vi "INI Input Clusters.vi"() -> (0 "File output directories":T2={"Archive Location"=path "", "Archive Location 2"=path "<Not A Path>", "OutPut Path"=path "", "Directory(s) To Scan Files"=[]}, 1 "FTP CRED Cluster":T4={"Host"="", "UserName"="", "PassWord"="", "FTP File Path"="", "FTP Timeout (S)"=60, "Active or Passive"=FALSE, "ASCII or Binary"=FALSE} {"FTP Timeout (S)" min=0 max=300 step=1}, 2 "Email Notification Cluster":T3={"Mail Server"="", "Return Address"="", "Email User Name"="", "Password"="", "Ping Address 1"="10.0.0.40", "Ping Address 2"="google.com", "Ping Address FTP Host"="web1026.ixwebhosting.com", "Ping address 1"=FALSE, "Ping address 2"=FALSE, "Ping FTP Host"=FALSE}, 3 "Email Recipiant List":string[](array[string]), 4 "error out":errorcluster, 5 "time stamp":timestamp, 6 "Site ID":string, 7 "File Management cluster":T1, 8 "Auto FTP":bool, 9 "Auto Archive":bool, 11 "hours old date mod(hours)":u8=2)   [LabVIEW 2011]
uses:
  Controls/FTP Credintials.ctl
  Controls/Ping address and email notify.ctl
  Controls/File Path directories.ctl
  Controls/File Management.ctl
  <vilib>/Utility/sysdir.llb/System Directory Type.ctl
  <vilib>/Utility/config.llb/Read Key (String).vi
  <vilib>/Utility/config.llb/Read Key (Boolean).vi
  <vilib>/Utility/config.llb/Read Key (Path).vi
  <vilib>/Utility/config.llb/Read Key (I32).vi
  <vilib>/Utility/config.llb/Read Key (U32).vi
  <vilib>/Utility/config.llb/NI_LVConfig.lvlib
panel:
  # "File Handling Method"
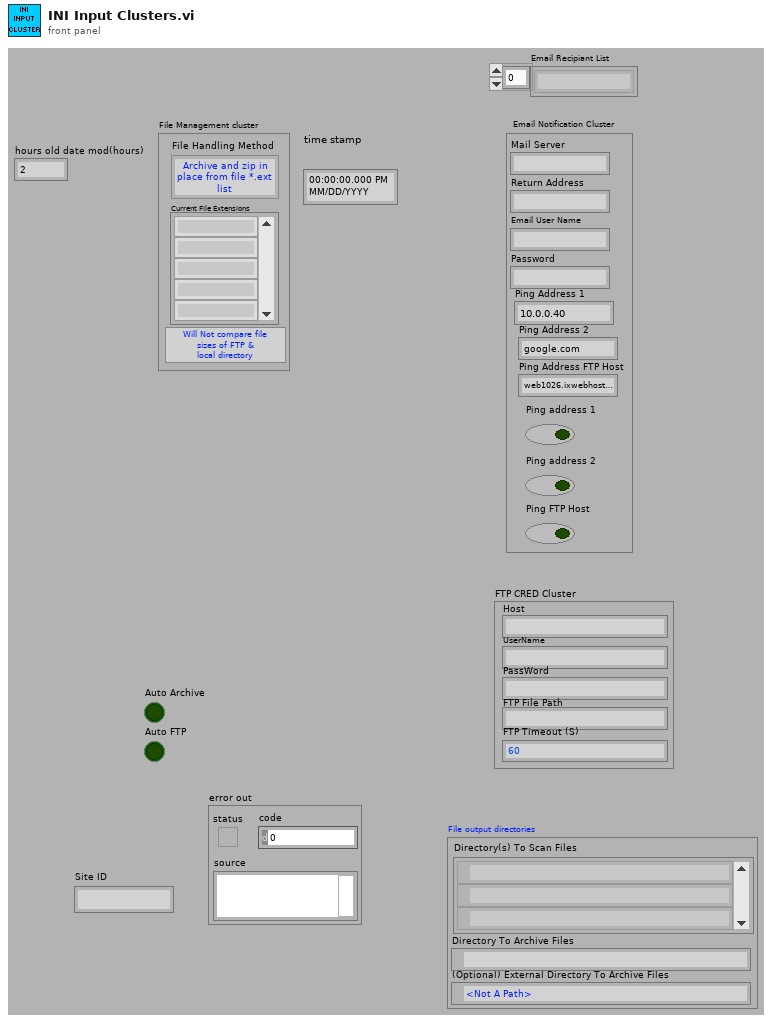
[diagram p1: front panel]
types:
  T1 = typedef "File Management.ctl" = cluster{"Comp File Size":bool, "File Handle Method":enum16{"Archive and zip in place from file *.ext list", "Archive and zip ALL file Types to archive directory", "Archive and zip to archive directory from file *.ext list", "Perform no file management"}, "file extention list":string[]}
  T2 = typedef "File Path directories.ctl" = cluster{"Archive Location":path, "Archive Location 2":path, "OutPut Path":path, "Directory(s) To Scan Files":path[]}
  T3 = typedef "Ping address and email notify.ctl" = cluster{"Mail Server":string, "Return Address":string, "Email User Name":string, "Password":string, "Ping Address 1":string, "Ping Address 2":string, "Ping Address FTP Host":string, "Ping address 1":bool, "Ping address 2":bool, "Ping FTP Host":bool}
  T4 = typedef "FTP Credintials.ctl" = cluster{"Host":string, "UserName":string, "PassWord":string, "FTP File Path":string, "FTP Timeout (S)":i32, "Active or Passive":bool, "ASCII or Binary":bool}
  T5 = enum16{"Archive and Zip IN Place", "Archive and Zip All File Types", "Archive and Zip from List of File Extensions ", "Perform No File Management"}
  T6 = typedef "System Directory Type.ctl" = i32
  T7 = typedef "NI_LVConfig.lvlib/Config Data RefNum.ctl" = refnum<k1>
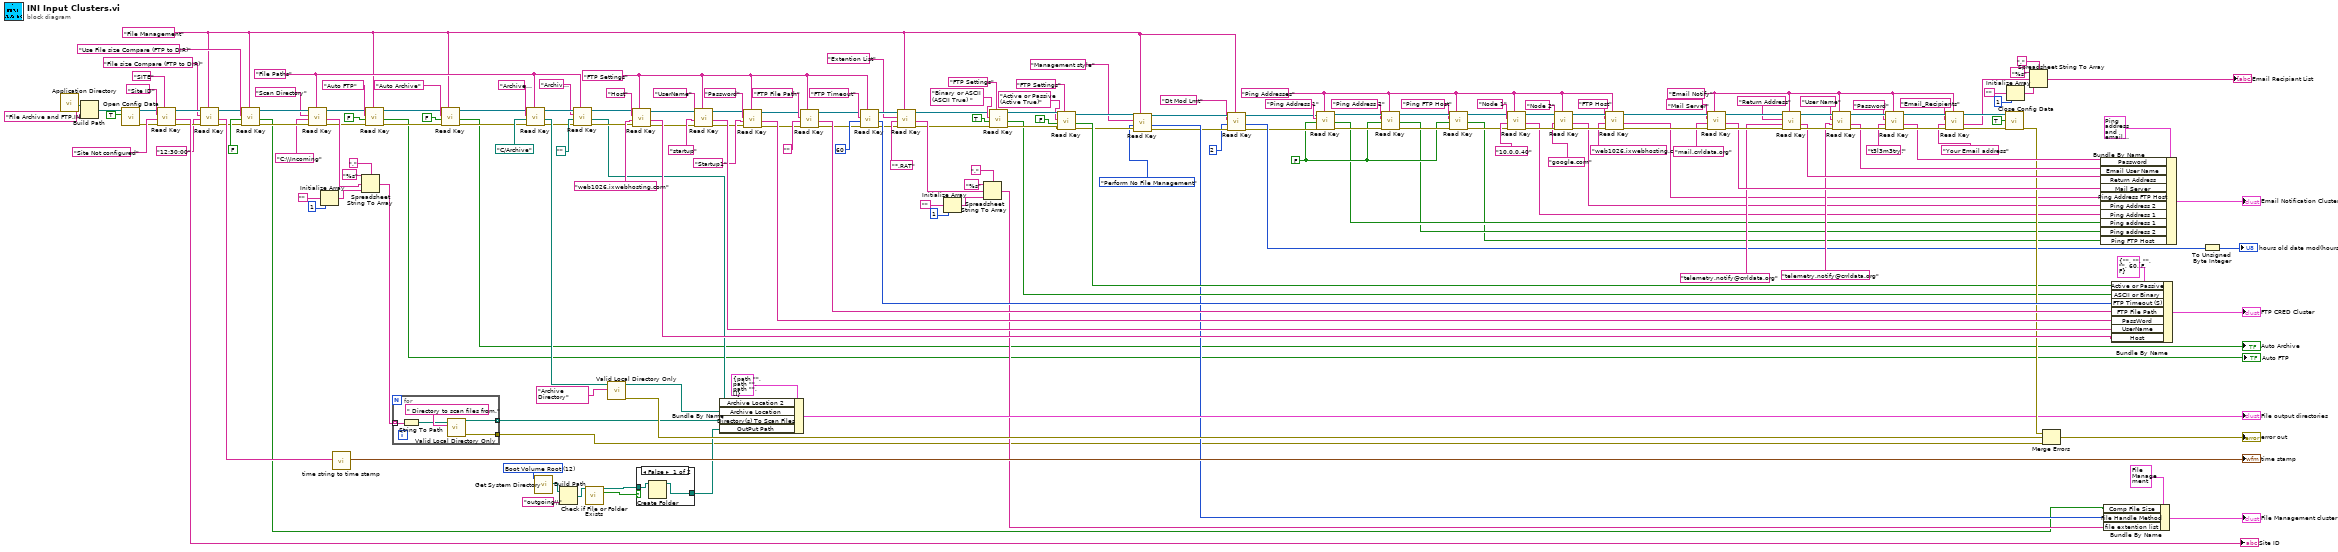
[diagram p0: block diagram]
diagram:
  w4 = FALSE
  w30 = "File Management" ("section")
  w80 = T6 12 items=["User Home"=0, "User Desktop"=1, "User Documents"=2, "User Application Data"=3, "User Preferences"=4, "User Temporary"=5, "Public Documents"=6, "Public Application Data"=7, "Public Preferences"=8, "Public Cache"=13, "System Core Libraries"=9, "System Installed Libraries"=10, "Application Files"=11, "Boot Volume Root"=12] ("system directory type")
  w108 = "FTP Settings" ("name or relative path")
  w97 = "File Paths" ("name or relative path")
  w5 = "Ping Addresses" ("name or relative path")
  w198 = "Email Notify" ("name or relative path")
  n1 = call <vilib>:"Application Directory.vi"() -> ("Application Directory"=w19:path)
  n2 = Build Path(base path=w19, name or relative path="File Archive and FTP.INI") -> (appended path=w146:path)
  n3 = call <vilib>:"Open Config Data.vi"("create file if necessary (T)"=TRUE, "configuration file path"=w146) -> ("error out"=w135:errorcluster, "refnum"=w136:T7)  [unwired: 7 in, 1 out]
  n4 = call-poly <vilib>:"Read Key.vi"("section"="SITE" ("name or relative path"), "error in (no error)"=w135, "default value"="Site Not configured", "key"="Site ID" ("name or relative path"), "refnum"=w136) -> ("error out"=w138:errorcluster, "value"=→"Site ID":string, "refnum out"=w137:T7)  [unwired: 3 in, 1 out]
  n5 = call-poly <vilib>:"Read Key.vi"("section"=w30, "error in (no error)"=w138, "default value"="12:30:00", "key"="File size Compare (FTP to DIR)" ("name or relative path"), "refnum"=w137) -> ("error out"=w126:errorcluster, "value"=w133:string, "refnum out"=w127:T7)  [unwired: 3 in, 1 out]
  n6 = call-poly <vilib>:"Read Key.vi"("section"=w30, "error in (no error)"=w126, "default value"=FALSE ("create file if necessary (T)"), "key"="Use File size Compare (FTP to DIR)" ("name or relative path"), "refnum"=w127) -> ("error out"=w129:errorcluster, "value"=w53:bool, "refnum out"=w128:T7)  [unwired: 3 in, 1 out]
  n7 = call-poly <vilib>:"Read Key.vi"("section"=w97, "error in (no error)"=w129, "default value"="C:\\Incoming", "key"="Scan Directory" ("name or relative path"), "refnum"=w128) -> ("error out"=w26:errorcluster, "value"=w42:string, "refnum out"=w29:T7)  [unwired: 3 in, 1 out]
  n8 = Initialize Array("", 1 ("dimension size")) -> (w43:string[])
  n9 = call "time string to time stamp.vi"("time string example(16:15:00)"=w133) -> ("time stamp"=→"time stamp":timestamp)  [unwired: 10 in]
  n10 = Spreadsheet String To Array(delimiter (Tab)=",", format string="%s", spreadsheet string=w42, array type (2D Dbl)=w43) -> (array=w41:string[])
  n11 = call-poly <vilib>:"Read Key.vi"("section"=w30, "error in (no error)"=w26, "default value"=FALSE, "key"="Auto FTP" ("name or relative path"), "refnum"=w29) -> ("error out"=w25:errorcluster, "value"=→"Auto FTP":bool, "refnum out"=w28:T7)  [unwired: 3 in, 1 out]
  n12 = for {
    tunnel: w41 -> [w205] mode=indexing
    tunnel: [w202] -> w40 mode=indexing
    tunnel: [w201] -> w39
    n13 = String To Path(string=w205) -> (path=w203:path)
    n14 = call "Valid Local Directory Only.vi"("Directory ref"=" Directory to scan files from.", "Path input"=w203) -> ("error out"=w201:errorcluster, "Path output"=w202:path)  [unwired: 8 in]
  }
  n15 = call-poly <vilib>:"Read Key.vi"("section"=w30, "error in (no error)"=w25, "default value"=FALSE, "key"="Auto Archive" ("name or relative path"), "refnum"=w28) -> ("error out"=w24:errorcluster, "value"=→"Auto Archive":bool, "refnum out"=w27:T7)  [unwired: 3 in, 1 out]
  n16 = call-poly <vilib>:"Read Key.vi"("section"=w97, "error in (no error)"=w24, "default value"=path "C:/Archive", "key"="Archive location 1" ("name or relative path"), "refnum"=w27) -> ("error out"=w95:errorcluster, "value"=w144:path, "refnum out"=w94:T7)  [unwired: 3 in, 1 out]
  n17 = call <vilib>:"Get System Directory.vi"("system directory type"=w80) -> ("system directory"=w79:path)  [unwired: 10 in]
  n18 = Build Path(base path=w79, name or relative path="outgoing\\") -> (appended path=w82:path)
  n19 = call-poly <vilib>:"Read Key.vi"("section"=w97, "error in (no error)"=w95, "default value"=path "", "key"="Archive location 2" ("name or relative path"), "refnum"=w94) -> ("error out"=w98:errorcluster, "value"=w91:path, "refnum out"=w103:T7)  [unwired: 3 in, 1 out]
  n20 = call <vilib>:"Check if File or Folder Exists.vi"("path"=w82) -> ("file or folder exists?"=w78:bool, "dup path"=w77:path)  [unwired: 8 in, 1 out]
  n21 = call "Valid Local Directory Only.vi"("Directory ref"="Archive Directory", "Path input"=w144) -> ("error out"=w147:errorcluster, "Path output"=w87:path)  [unwired: 8 in]
  n22 = call-poly <vilib>:"Read Key.vi"("section"=w108, "error in (no error)"=w98, "default value"="web1026.ixwebhosting.com" ("name or relative path"), "key"="Host" ("name or relative path"), "refnum"=w103) -> ("error out"=w99:errorcluster, "value"=w134:string, "refnum out"=w104:T7)  [unwired: 3 in, 1 out]
  n23 = case shown="False" w78 {
    tunnel: w77 -> [w207 w208]
    tunnel: [w206 w208] -> w76
    frame False {
      n24 = Create Folder(path (use dialog)=w207) -> (created path=w206:path)  [unwired: 2 in, 2 out]
    }
    frame True {
    }
  }
  n25 = call-poly <vilib>:"Read Key.vi"("section"=w108, "error in (no error)"=w99, "default value"="startup" ("name or relative path"), "key"="UserName" ("name or relative path"), "refnum"=w104) -> ("error out"=w100:errorcluster, "value"=w123:string, "refnum out"=w105:T7)  [unwired: 3 in, 1 out]
  n26 = Bundle By Name(cluster=T2 {"Archive Location"=path "", "Archive Location 2"=path "", "OutPut Path"=path "", "Directory(s) To Scan Files"=[]} ("File Path Array"), "Archive Location 2"=w91, "Archive Location"=w87, "Directory(s) To Scan Files"=w40, "OutPut Path"=w76) -> (→"File output directories":T2)
  n27 = call-poly <vilib>:"Read Key.vi"("section"=w108, "error in (no error)"=w100, "default value"="Startup1" ("name or relative path"), "key"="Password" ("name or relative path"), "refnum"=w105) -> ("error out"=w101:errorcluster, "value"=w122:string, "refnum out"=w106:T7)  [unwired: 3 in, 1 out]
  n28 = call-poly <vilib>:"Read Key.vi"("section"=w108, "error in (no error)"=w101, "default value"="" ("name or relative path"), "key"="FTP File Path" ("name or relative path"), "refnum"=w106) -> ("error out"=w102:errorcluster, "value"=w121:string, "refnum out"=w107:T7)  [unwired: 3 in, 1 out]
  n29 = call-poly <vilib>:"Read Key.vi"("section"=w108, "error in (no error)"=w102, "default value"=60, "key"="FTP Timeout" ("name or relative path"), "refnum"=w107) -> ("error out"=w66:errorcluster, "value"=w148:i32, "refnum out"=w65:T7)  [unwired: 3 in, 1 out]
  n30 = call-poly <vilib>:"Read Key.vi"("section"=w30, "error in (no error)"=w66, "default value"="*.RAT", "key"="Extention List", "refnum"=w65) -> ("error out"=w64:errorcluster, "value"=w68:string, "refnum out"=w63:T7)  [unwired: 3 in, 1 out]
  n31 = Initialize Array("", 1 ("dimension size")) -> (w73:string[])
  n32 = Spreadsheet String To Array(delimiter (Tab)=",", format string="%s", spreadsheet string=w68, array type (2D Dbl)=w73) -> (array=w59:string[])
  n33 = call-poly <vilib>:"Read Key.vi"("section"="FTP Settings" ("name or relative path"), "error in (no error)"=w64, "default value"=TRUE, "key"="Binary or ASCII (ASCII True) " ("name or relative path"), "refnum"=w63) -> ("error out"=w200:errorcluster, "value"=w75:bool, "refnum out"=w199:T7)  [unwired: 3 in, 1 out]
  n34 = call-poly <vilib>:"Read Key.vi"("section"="FTP Settings" ("name or relative path"), "error in (no error)"=w200, "default value"=FALSE, "key"="Active or Passive (Active True)" ("name or relative path"), "refnum"=w199) -> ("error out"=w57:errorcluster, "value"=w74:bool, "refnum out"=w58:T7)  [unwired: 3 in, 1 out]
  n35 = call-poly <vilib>:"Read Key.vi"("section"=w30, "error in (no error)"=w57, "default value"=T5."Perform No File Management" ("File Handle Method"), "key"="Management style", "refnum"=w58) -> ("error out"=w37:errorcluster, "value"=w55:i32, "refnum out"=w38:T7)  [unwired: 3 in, 1 out]
  n36 = call-poly <vilib>:"Read Key.vi"("section"=w30, "error in (no error)"=w37, "default value"=u32 2, "key"="Dt Mod Lmt" ("name or relative path"), "refnum"=w38) -> ("error out"=w11:errorcluster, "value"=w34:u32, "refnum out"=w15:T7)  [unwired: 3 in, 1 out]
  n37 = call-poly <vilib>:"Read Key.vi"("section"=w5, "error in (no error)"=w11, "default value"=w4, "key"="Ping Address 1" ("Mail Server"), "refnum"=w15) -> ("error out"=w10:errorcluster, "value"=w3:bool, "refnum out"=w14:T7)  [unwired: 3 in, 1 out]
  n38 = call-poly <vilib>:"Read Key.vi"("section"=w5, "error in (no error)"=w10, "default value"=w4, "key"="Ping Address 2" ("Mail Server"), "refnum"=w14) -> ("error out"=w9:errorcluster, "value"=w2:bool, "refnum out"=w13:T7)  [unwired: 3 in, 1 out]
  n39 = call-poly <vilib>:"Read Key.vi"("section"=w5, "error in (no error)"=w9, "default value"=w4, "key"="Ping FTP Host" ("Mail Server"), "refnum"=w13) -> ("error out"=w8:errorcluster, "value"=w1:bool, "refnum out"=w12:T7)  [unwired: 3 in, 1 out]
  n40 = call-poly <vilib>:"Read Key.vi"("section"=w5, "error in (no error)"=w8, "default value"="10.0.0.40", "key"="Node 1" ("Mail Server"), "refnum"=w12) -> ("error out"=w169:errorcluster, "value"=w84:string, "refnum out"=w168:T7)  [unwired: 3 in, 1 out]
  n41 = call-poly <vilib>:"Read Key.vi"("section"=w5, "error in (no error)"=w169, "default value"="google.com", "key"="Node 2" ("Mail Server"), "refnum"=w168) -> ("error out"=w170:errorcluster, "value"=w85:string, "refnum out"=w171:T7)  [unwired: 3 in, 1 out]
  n42 = call-poly <vilib>:"Read Key.vi"("section"=w5, "error in (no error)"=w170, "default value"="web1026.ixwebhosting.com", "key"="FTP Host" ("Mail Server"), "refnum"=w171) -> ("error out"=w173:errorcluster, "value"=w86:string, "refnum out"=w172:T7)  [unwired: 3 in, 1 out]
  n43 = call-poly <vilib>:"Read Key.vi"("section"=w198, "error in (no error)"=w173, "default value"="mail.crrldata.org", "key"="Mail Server" ("Mail Server"), "refnum"=w172) -> ("error out"=w180:errorcluster, "value"=w161:string, "refnum out"=w181:T7)  [unwired: 3 in, 1 out]
  n44 = call-poly <vilib>:"Read Key.vi"("section"=w198, "error in (no error)"=w180, "default value"="telemetry.notify@crrldata.org", "key"="Return Address" ("Return Address"), "refnum"=w181) -> ("error out"=w182:errorcluster, "value"=w160:string, "refnum out"=w185:T7)  [unwired: 3 in, 1 out]
  n45 = call-poly <vilib>:"Read Key.vi"("section"=w198, "error in (no error)"=w182, "default value"="telemetry.notify@crrldata.org", "key"="User Name" ("Email User Name"), "refnum"=w185) -> ("error out"=w183:errorcluster, "value"=w159:string, "refnum out"=w184:T7)  [unwired: 3 in, 1 out]
  n46 = call-poly <vilib>:"Read Key.vi"("section"=w198, "error in (no error)"=w183, "default value"="t3l3m3try!", "key"="Password" ("Password"), "refnum"=w184) -> ("error out"=w194:errorcluster, "value"=w158:string, "refnum out"=w193:T7)  [unwired: 3 in, 1 out]
  n47 = call-poly <vilib>:"Read Key.vi"("section"=w198, "error in (no error)"=w194, "default value"="Your Email address", "key"="Email_Recipients" ("Password"), "refnum"=w193) -> ("error out"=w197:errorcluster, "value"=w195:string, "refnum out"=w196:T7)  [unwired: 3 in, 1 out]
  n48 = call <vilib>:"Close Config Data.vi"("error in (no error)"=w197, "write file if changed (T)"=TRUE, "refnum"=w196) -> ("error out"=w90:errorcluster)  [unwired: 7 in, 1 out]
  n49 = Initialize Array("", 1 ("dimension size")) -> (w186:string[])
  n50 = Spreadsheet String To Array(delimiter (Tab)=",", format string="%s", spreadsheet string=w195, array type (2D Dbl)=w186) -> (array=→"Email Recipiant List":string[])
  n51 = Merge Errors(w90, w147, w39) -> (→"error out":errorcluster)
  n52 = Bundle By Name(cluster=T3 {"Mail Server"="mail.crrldata.org", "Return Address"="telemetry.notify@crrldata.org", "Email User Name"="telemetry.notify@crrldata.org", "Password"="t3l3m3try!", "Ping Address 1"="10.0.0.40", "Ping Address 2"="google.com", "Ping Address FTP Host"="web1026.ixwebhosting.com", "Ping address 1"=FALSE, "Ping address 2"=FALSE, "Ping FTP Host"=FALSE} ("Email Notification Cluster"), "Password"=w158, "Email User Name"=w159, "Return Address"=w160, "Mail Server"=w161, "Ping Address FTP Host"=w86, "Ping Address 2"=w85, "Ping Address 1"=w84, "Ping address 1"=w3, "Ping address 2"=w2, "Ping FTP Host"=w1) -> (→"Email Notification Cluster":T3)
  n53 = Bundle By Name(cluster=T1 {"Comp File Size"=FALSE, "File Handle Method"=enum."Archive and zip in place from file *.ext list", "file extention list"=[]} ("File Management"), "Comp File Size"=w53, "File Handle Method"=w55, "file extention list"=w59) -> (→"File Management cluster":T1)
  n54 = Bundle By Name(cluster=T4 {"Host"="", "UserName"="", "PassWord"="", "FTP File Path"="", "FTP Timeout (S)"=60, "Active or Passive"=FALSE, "ASCII or Binary"=FALSE} ("FTP Creds"), "Active or Passive"=w74, "ASCII or Binary"=w75, "FTP Timeout (S)"=w148, "FTP File Path"=w121, "PassWord"=w122, "UserName"=w123, "Host"=w134) -> (→"FTP CRED Cluster":T4)
  n55 = To Unsigned Byte Integer(number=w34) -> (unsigned 8bit integer=→"hours old date mod(hours)":u8)
